vi "Handle Control Request.vi"(8 "error in (no error)":errorcluster, 10 "Command Requester":T1, 11 "RDS Controller Actor in":refnum<class "RDS Controller Actor.lvclass">) -> (0 "error out":errorcluster, 3 "RDS Controller Actor out":refnum<class "RDS Controller Actor.lvclass">)   [LabVIEW 2015, in "RDS Controller Actor.lvlib" / "RDS Controller Actor.lvclass"]
uses:
  RDS Controller Actor.lvclass
  Controller.ctl
  Libraries/RDS Child Messages/Controller Message/Controller Message.lvclass
  Libraries/RDS Framework/RDS Message ID.ctl
  Libraries/RDS Child Messages/Controller Message/Controller Message Type.ctl
  RDS Controller Actor.lvclass/RDS Controller Actor.ctl
  Libraries/RDS Framework/RDS Message Class/RDS Message.lvclass/RDS Message.ctl
  Libraries/RDS Child Messages/Controller Message/Controller Message.lvclass/Controller Message.ctl
  Libraries/RDS Framework/RDS Message Class/RDS Message.lvclass
  Libraries/RDS Child Messages/RDS Child Messages.lvlib
  RDS Parent Actor/RDS Parent Actor/RDS Parent Actor.lvclass
  RDS Helm Actor/RDS Helm Actor.lvlib
  RDS Controller Actor.lvlib
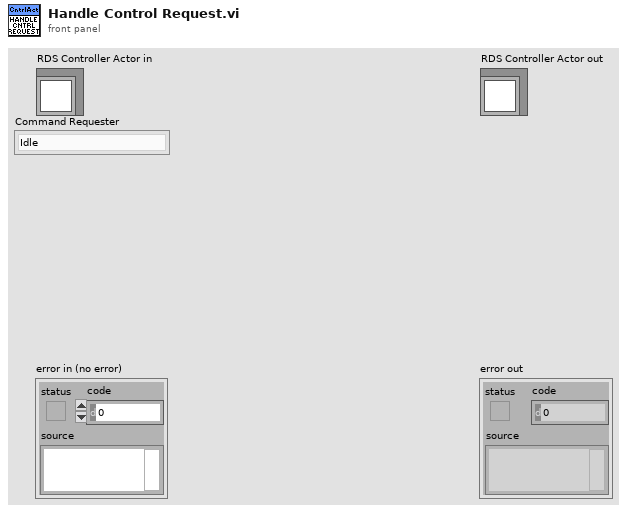
[diagram p1: front panel]
types:
  T1 = typedef "RDS Controller Actor.lvlib/Controller.ctl" = enum16{"Idle", "Local Remote Control", "Shore Remote Control", "Mission Control"}
  T2 = typedef "RDS Child Messages.lvlib/Controller Message.lvclass/Controller Message Type.ctl" = enum16{"Control Relinquish Request", "Control Relinquish Command", "Control Request", "Control Granted"}
  T3 = typedef "RDS Child Messages.lvlib/RDS Message ID.ctl" = enum16{"RDS Hello World", "String Message", "AIP_Status", "AIP_Command", "GPS_Data", "MCB_Command", "MCB_Status", "Compass_Data", "Depth_Data", "Battery_Data", "Contoller_State", "Set_Mag_Dev", "BTB_Shutdown", "State_Sample_Request", "State_Sample", "PID_Gains_Set", "Helm_Limiter_Set", "Helm_Heading_Command", "Helm_Steering_Command", "Helm_Status", "Controller_Message", "AIP_Set_Min_Depth", "Mission_Controller_State", "Mission_Upload", "Mission_Set_Op_and_Run", "Mission_Settings_Set"}
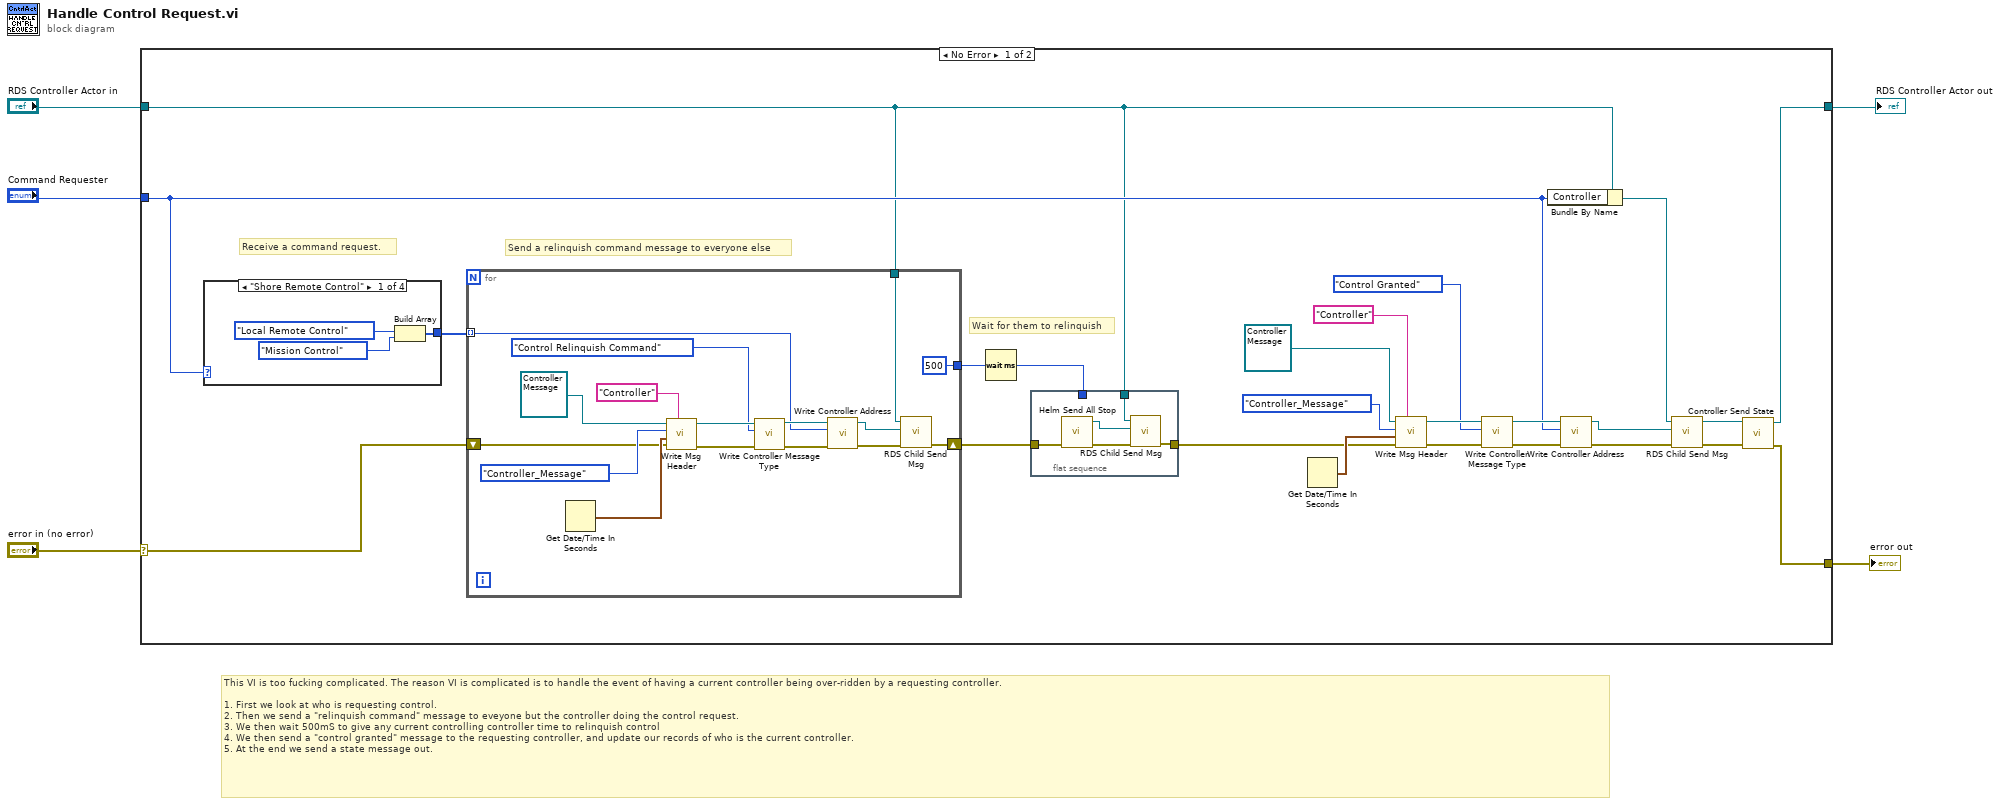
[diagram p0: block diagram]
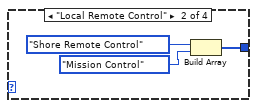
[diagram p2: hidden frame]
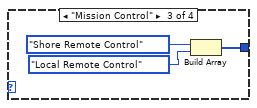
[diagram p3: hidden frame]
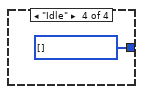
[diagram p4: hidden frame]
diagram:
  # "This VI is too fucking complicated. The reason VI is complicated is to handle the event of having a current controller being over-ridden by a requesting controller.\n\n1. First we look at who is requesting control.\n2. Then we send a \"relinquish command\" message to eveyone but the controller doing the control request.\n3. We then wait 500mS to give any current controlling controller time to relinquish control\n4. We then send a \"control granted\" message to the requesting controller, and update our records of who is the current controller.\n5. At the end we send a state message out."
  n1 = case shown="No Error" "error in (no error)" {
    selector: "error in (no error)" -> [w6 w62]
    tunnel: [w7 w62] -> w4
    tunnel: [w11 w61] -> w2
    tunnel: "RDS Controller Actor in" -> [w15 w61]
    tunnel: "Command Requester" -> [w16 _]
    frame No Error {
      # "Wait for them to relinquish"
      # "Send a relinquish command message to everyone else"
      # "Receive a command request."
      n2 = case shown="\"Shore Remote Control\"" w16 {
        tunnel: [w51 w54 w57 w60] -> w14
        frame "Shore Remote Control" {
          n3 = Build Array(Controller."Local Remote Control" ("Command Requester"), Controller."Mission Control" ("Command Requester")) -> (w51:T1[])
        }
        frame "Local Remote Control" {
          n4 = Build Array(Controller."Shore Remote Control" ("Command Requester"), Controller."Mission Control" ("Command Requester")) -> (w54:T1[])
        }
        frame "Mission Control" {
          n5 = Build Array(Controller."Shore Remote Control" ("Command Requester"), Controller."Local Remote Control" ("Command Requester")) -> (w57:T1[])
        }
        frame "Idle" {
          w60 = T1[] [] items=["Idle", "Local Remote Control", "Shore Remote Control", "Mission Control"]
        }
      }
      n6 = for {
        tunnel: w15 -> [w40]
        tunnel: [u32 500 ("milliseconds to wait")] -> w20
        tunnel: w14 -> [w37] mode=indexing
        shift-right: [w39] -> w19
        shift-left: w6 -> [w35]
        n7 = Get Date/Time In Seconds() -> (seconds since 1Jan1904=w47:timestamp)
        n8 = call "Write Msg Header.vi"("Sender Name"="Controller", "error in (no error)"=w35, "Time Stamp"=w47, "Msg ID"=RDS_Message_ID."Controller_Message", "RDS Message in"=refnum<class "Controller Message.lvclass"> refnum ("RDS Child Messages.lvlib:Controller Message.lvclass")) -> ("error out"=w46:errorcluster, "RDS Message out"=w45:refnum<class "Controller Message.lvclass">)  [unwired: 5 in]
        n9 = call "Write Controller Message Type.vi"("error in (no error)"=w46, "Controller Message Type"=Controller_Message_Type."Control Relinquish Command", "Controller Message in"=w45) -> ("error out"=w42:errorcluster, "Controller Message out"=w43:refnum<class "Controller Message.lvclass">)  [unwired: 7 in]
        n10 = call "Write Controller Address.vi"("error in (no error)"=w42, "Controller"=w37, "Controller Message in"=w43) -> ("error out"=w41:errorcluster, "Controller Message out"=w36:refnum<class "Controller Message.lvclass">)  [unwired: 7 in]
        n11 = call "RDS Child Send Msg.vi"("error in (no error)"=w41, "RDS Message"=w36, "RDS Parent Actor in"=w40) -> ("error out"=w39:errorcluster)  [unwired: 7 in, 1 out]
      }
      n12 = Wait (ms)(milliseconds to wait=w20) -> (millisecond timer value=w18:u32)
      n13 = flat-sequence {
        tunnel: w19 -> [w34]
        tunnel: w18 -> [_]
        tunnel: [w32] -> w17
        tunnel: w15 -> [w30]
        frame #0 {
          n14 = call "Helm Send All Stop.vi"("error in (no error)"=w34) -> ("error out"=w33:errorcluster, "All Stop Message"=w31:refnum<class "Steering Command.lvclass">)  [unwired: 9 in]
          n15 = call "RDS Child Send Msg.vi"("error in (no error)"=w33, "RDS Message"=w31, "RDS Parent Actor in"=w30) -> ("error out"=w32:errorcluster)  [unwired: 7 in, 1 out]
        }
      }
      n16 = Get Date/Time In Seconds() -> (seconds since 1Jan1904=w29:timestamp)
      n17 = call "Write Msg Header.vi"("Sender Name"="Controller", "error in (no error)"=w17, "Time Stamp"=w29, "Msg ID"=RDS_Message_ID."Controller_Message", "RDS Message in"=refnum<class "Controller Message.lvclass"> refnum ("RDS Child Messages.lvlib:Controller Message.lvclass")) -> ("error out"=w21:errorcluster, "RDS Message out"=w25:refnum<class "Controller Message.lvclass">)  [unwired: 5 in]
      n18 = call "Write Controller Message Type.vi"("error in (no error)"=w21, "Controller Message Type"=Controller_Message_Type."Control Granted", "Controller Message in"=w25) -> ("error out"=w22:errorcluster, "Controller Message out"=w23:refnum<class "Controller Message.lvclass">)  [unwired: 7 in]
      n19 = Bundle By Name(cluster=w15, "Controller"=w16) -> (w10:refnum<class "RDS Controller Actor.lvclass">)
      n20 = call "Write Controller Address.vi"("error in (no error)"=w22, "Controller"=w16, "Controller Message in"=w23) -> ("error out"=w13:errorcluster, "Controller Message out"=w12:refnum<class "Controller Message.lvclass">)  [unwired: 7 in]
      n21 = call "RDS Child Send Msg.vi"("error in (no error)"=w13, "RDS Message"=w12, "RDS Parent Actor in"=w10) -> ("error out"=w8:errorcluster, "RDS Parent Actor out"=w9:refnum<class "RDS Controller Actor.lvclass">)  [unwired: 7 in]
      n22 = call "Controller Send State.vi"("error in (no error)"=w8, "RDS Controller Actor in"=w9) -> ("error out"=w7:errorcluster, "RDS Controller Actor out"=w11:refnum<class "RDS Controller Actor.lvclass">)  [unwired: 8 in]
    }
    frame Error {
    }
  }
  "error out" <- w4
  "RDS Controller Actor out" <- w2
